vi "UI_Update_Status.vi"(8 "error in (no error)":errorcluster caption="entrée d'erreur (pas d'erreur)", 10 "UI Status":T4, 11 "QMH UI Cluster":T1) -> (0 "error out":errorcluster caption="sortie d'erreur", 2 "Variant":variant, 3 "QMH UI Cluster":T1)   [LabVIEW 2020]
doc: "This VI updates the UI and ICR Status according to the User action.\nIt stores the status values into the UI Report and updates the indicator PIL Status."
uses:
  controls/QMH_UI_Cluster.ctl
  controls/QMH_UI_References.ctl
  controls/QMH_UI_Report.ctl
  controls/QMH_UI_Command.ctl
  controls/QMH_ICR_Command.ctl
  controls/QMH_Status.ctl
  controls/PIL_Status.ctl
panel:
  in  "PIL Status":T7
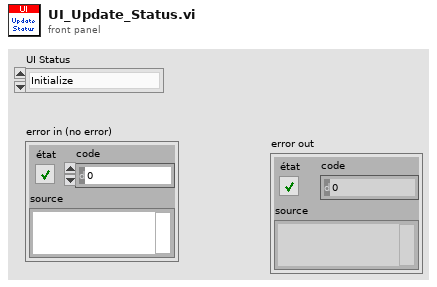
[diagram p1: front panel]
types:
  T1 = typedef "QMH_UI_Cluster.ctl" = cluster{"QMH UI References":T2, "QMH UI Report":T3}
  T2 = typedef "QMH_UI_References.ctl" = cluster{"Refnum Load":refnum<vi>, "Refnum Save As":refnum<vi>, "Refnum Start":refnum<vi>, "Refnum Exit":refnum<vi>, "Refnum Tabs":refnum<vi>, "Refnum SPECTRUM":refnum<vi>, "Refnum EXPERIMENT":refnum<vi>, "Refnum VOLTAGES":refnum<vi>, "Refnum SEQUENCE":refnum<vi>, "Refnum EXPERT":refnum<vi>, "Refnum LOOPS":refnum<vi>, "Refnum EXCIT Table":refnum<vi>, "Refnum TIMING Table":refnum<vi>, "Refnum CHANGE Experiment":refnum<vi>, "Refnum CHANGE Voltages":refnum<vi>, "Refnum CHANGE Sequence":refnum<vi>, "Refnum CHANGE Expert":refnum<vi>, "Refnum CHANGE Scientist":refnum<vi>, "Refnum PIL Status":refnum<vi>}
  T3 = typedef "QMH_UI_Report.ctl" = cluster{"UI Status":T4, "ICR Status":T5, "QMH Status":T6}
  T4 = typedef "QMH_UI_Command.ctl" = enum16{"Initialize", "UI Load", "UI Save", "UI Save As", "UI Change Experiment", "UI Change Voltages", "UI Change Sequence", "UI Change Expert", "UI Change Loops", "UI Change Scientist", "Ready to Start", "UI Start", "Waiting for ICR", "UI Exit", "Update Experiment", "Update Report", "Update ICR Status", "Waiting for User"}
  T5 = typedef "QMH_ICR_Command.ctl" = enum16{"Initialize", "Sequence Loop Setup", "Sequence Setup", "ICR Start", "ICR Stop", "Hardware Setup", "Next Sequence Loop", "Next Accumulation", "Waiting for Trigger", "Sequence Started", "Sequence Finished", "Sequence Loop Done", "Writing Data", "Hardware Reset", "Exit"}
  T6 = typedef "QMH_Status.ctl" = enum16{"Init", "Loading", "Setup", "Ready to Start", "Started", "Idle"}
  T7 = typedef "PIL_Status.ctl" = cluster{"UI Status":string, "ICR Status":string, "QMH Status":string}
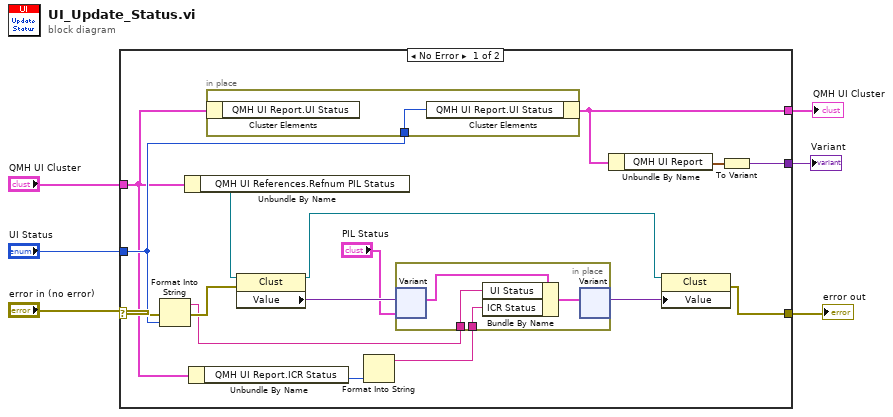
[diagram p0: block diagram]
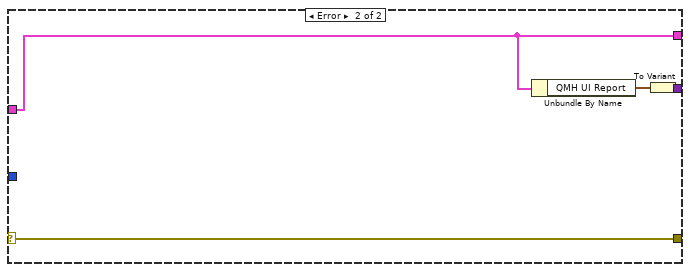
[diagram p2: hidden frame]
diagram:
  n1 = case shown="No Error" "error in (no error)" {
    selector: "error in (no error)" -> [w20 w31]
    tunnel: [w21 w31] -> w5
    tunnel: "UI Status" -> [w17 _]
    tunnel: "QMH UI Cluster" -> [w13 w30]
    tunnel: [w16 w30] -> w2
    tunnel: [w14 w29] -> w1
    frame No Error {
      n2 = Format Into String ("Format to String")(error in=w20, w17) -> (resulting string=w8:string, error out=w18:errorcluster)  [unwired: 2 in]
      n3 = Unbundle By Name(w13) -> ("QMH UI References.Refnum PIL Status"=w22:refnum<vi>)
      n4 = Unbundle By Name(w13) -> ("QMH UI Report.ICR Status"=w12:T5)
      n5 = in-place {
        in-place-border: w17 -> [w27]
        n6 = in-place-cluster #1(w13) -> ()  [unwired: 1 out]
        n7 = in-place-cluster #1("QMH UI Report.UI Status"=w27) -> (w16:T1)
      }
      n8 = property class="Clust"(reference=w22, error in=w18) -> (reference out=w19:refnum<vi>, "Value"=w11:variant)  [unwired: 1 out]
      n9 = Format Into String ("Format to String")(w12) -> (resulting string=w9:string)  [unwired: 3 in, 1 out]
      n10 = in-place {
        in-place-border: w9 -> [w25]
        in-place-border: w8 -> [w24]
        n11 = in-place-variant #2(w11, "PIL Status") -> (w26:T7)  [unwired: 1 out]
        n12 = Bundle By Name(cluster=w26, "UI Status"=w24, "ICR Status"=w25) -> (w23:T7)
        n13 = in-place-variant #2(w23) -> (w7:variant)  [unwired: 1 out]
      }
      n14 = Unbundle By Name(w16) -> ("QMH UI Report"=w15:T3)
      n15 = property class="Clust"(reference=w19, "Value"=w7) -> (error out=w21:errorcluster)  [unwired: 1 in, 1 out]
      n16 = To Variant(anything=w15) -> (Variant=w14:variant)
    }
    frame Error {
      n17 = Unbundle By Name(w30) -> ("QMH UI Report"=w28:T3)
      n18 = To Variant(anything=w28) -> (Variant=w29:variant)
    }
  }
  "error out" <- w5
  "QMH UI Cluster" <- w2
  "Variant" <- w1
